vi "4 I16 Array Shifter.vi"(6 "Trig Offset":u8, 8 "Input Valid":bool, 10 "Start of Read":bool, 11 "Input Data":i16[](array[numeric])=[0, 0, 0, 0]) -> (0 "Output Data Valid":bool, 3 "Output Data":i16[](array[numeric]))   [LabVIEW 2011]
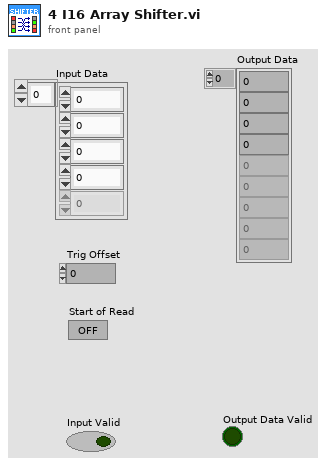
[diagram p1: front panel]
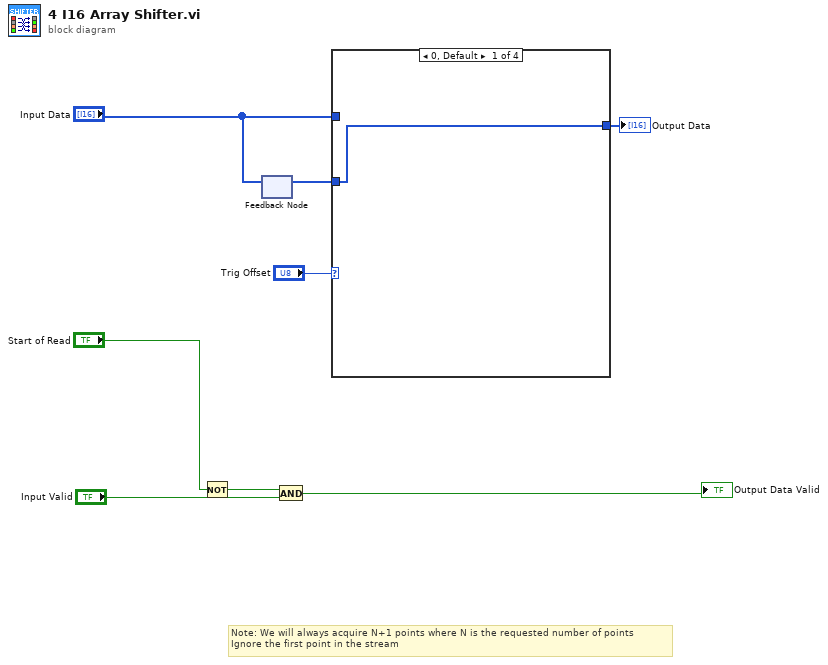
[diagram p0: block diagram]
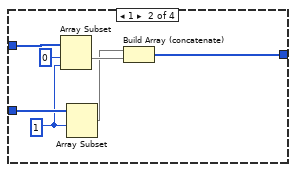
[diagram p2: hidden frame]
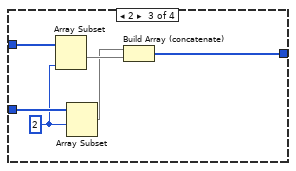
[diagram p3: hidden frame]
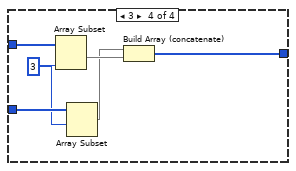
[diagram p4: hidden frame]
diagram:
  # "Note: We will always acquire N+1 points where N is the requested number of points\nIgnore the first point in the stream"
  n1 = Not(x="Start of Read") -> (.not. x?=w4:bool)
  n2 = feedback-in #1("Input Data") -> ()
  n3 = feedback #1() -> (w7:i16[])  [unwired: 1 in]
  n4 = And(x=w4, y="Input Valid") -> (x .and. y?=→"Output Data Valid":bool)
  n5 = case shown="0, Default" "Trig Offset" {
    tunnel: "Input Data" -> [_ w16 w22 w28]
    tunnel: w7 -> [w9 w15 w21 w27]
    tunnel: [w9 w12 w18 w24] -> w6
    frame 0, Default {
    }
    frame 1 {
      w11 = 1 ("index")
      n6 = Array Subset(array=w16, index=0, length=w11) -> (w14:i16[])
      n7 = Array Subset(array=w15, index=w11) -> (w13:i16[])  [unwired: 1 in]
      n8 = Build Array (concatenate)(w13, w14) -> (w12:i16[])
    }
    frame 2 {
      w17 = 2 ("index")
      n9 = Array Subset(array=w22, length=w17) -> (w20:i16[])  [unwired: 1 in]
      n10 = Array Subset(array=w21, index=w17) -> (w19:i16[])  [unwired: 1 in]
      n11 = Build Array (concatenate)(w19, w20) -> (w18:i16[])
    }
    frame 3 {
      w23 = 3 ("index")
      n12 = Array Subset(array=w28, length=w23) -> (w26:i16[])  [unwired: 1 in]
      n13 = Array Subset(array=w27, index=w23) -> (w25:i16[])  [unwired: 1 in]
      n14 = Build Array (concatenate)(w25, w26) -> (w24:i16[])
    }
  }
  "Output Data" <- w6
